vi "str to int64array.vi"(2 "String":string) -> (6 "int64 array":i64[](array[numeric]))   [LabVIEW 2014, in "OPCUA XML(dev).lvlib"]
uses:
  OPCUA XML(dev).lvlib
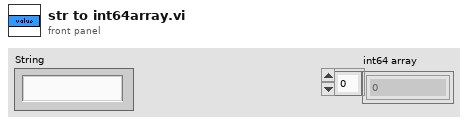
[diagram p1: front panel]
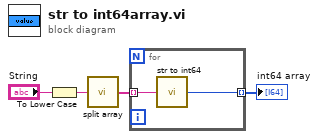
[diagram p0: block diagram]
diagram:
  n1 = To Lower Case(string="String") -> (all lower case string=w3:string)
  n2 = call "split array.vi"("string"=w3) -> ("split arr"=w2:string[])  [unwired: 8 in]
  n3 = for {
    tunnel: w2 -> [w6] mode=indexing
    tunnel: [w5] -> w1 mode=indexing
    n4 = call "str to int64.vi"("String"=w6) -> ("int64"=w5:i64)  [unwired: 6 in]
  }
  "int64 array" <- w1
